vi "Minimal AR Example.vi"() -> ()   [LabVIEW 2020, in "examples.lvlib"]
doc: "Demonstrate a minimal Augmented Reality Application which Captures from a Camera, Detects AprilTags and Overlays 3D Objects on the live Camera stream."
uses:
  examples.lvlib
  ar/tvec.ctl
  ar/Roll-Pitch-Yaw.ctl
  feature_detection/Apriltag Detector/Detector Settings.ctl
  capture/Stream/Stream.lvclass/Stream.ctl
  common/Camera Parameters.ctl
  common/Camera Matrix.ctl
  common/Camera Distortion Coefficients.ctl
  feature_detection/Apriltag Detector/AprilTag Detector.lvclass/AprilTag Detector.ctl
  image/ARGB Colour.ctl
  feature_detection/Apriltag Detector/Create (Tag36h11).vi
  image/New Image (Greyscale Preallocated).vi
  image/New Image (ARGB Preallocated).vi
  capture/Stream/Next Capture (ARGB).vi
  ar/Solve PnP (IPPE Square).vi
  image/Draw Filled Poly (ARGB).vi
  image/Draw Image to Picture (ARGB).vi
  image/New Image (Greyscale Preallocated).vi/6598b9e0-8a08-46f5-91fd-ca1b87217137.vi
  image/New Image (ARGB Preallocated).vi/3321fa97-f432-4e1e-8db9-a0df79aed21b.vi
  image/ARGB Colour to U32 Pixel Value.vi
  capture/Stream/Next Capture (ARGB).vi/66171ef0-1d22-3fc5-88a4-b174a611e83f.vi
  image/ARGBExtractChannel.vi
  ar/SolvePnPCore.vi
  ar/Build Square Marker Object Points.vi
  ar/Rodrigues.vi
  ar/Rodrigues (RVec To RMat).vi
  ar/Transform Components to Transformation Matrix.vi
  image/Draw Filled Poly (ARGB).vi/e24a04ad-8575-4d64-b8af-da4c51ecb9cd.vi
  ar/Project Points.vi
  image/Draw Line (ARGB).vi
  image/Draw Image to Picture (ARGB).vi/8cd07b1b-062e-4fe4-9e87-2eb3dc89fe0e.vi
  image/Draw Line (ARGB).vi/85aa1280-0fac-47da-ba54-33850455c996.vi
  feature_detection/Apriltag Detector/CreateDetector.vi
  <vilib>/Utility/error.llb/Error Cluster From Error Code.vi
  <vilib>/Analysis/Matrix/Numeric/Conversions/Array To Matrix.vi
  <vilib>/Analysis/Matrix/Numeric/Conversions/Array To Matrix - RA2.vi
  image/image.lvlib
  capture/capture.lvlib
  capture/Stream/Stream.lvclass
  common/common.lvlib
  feature_detection/Apriltag Detector/AprilTag Detector.lvclass
  ar/ar.lvlib
panel:
  in  "Rendering":enum16{"Project Points", "3D Engine"}(ring)
  in  "Stop":bool
  out "Picture":picture
  out "Poses":T3(array[cluster]) caption="Marker Poses"
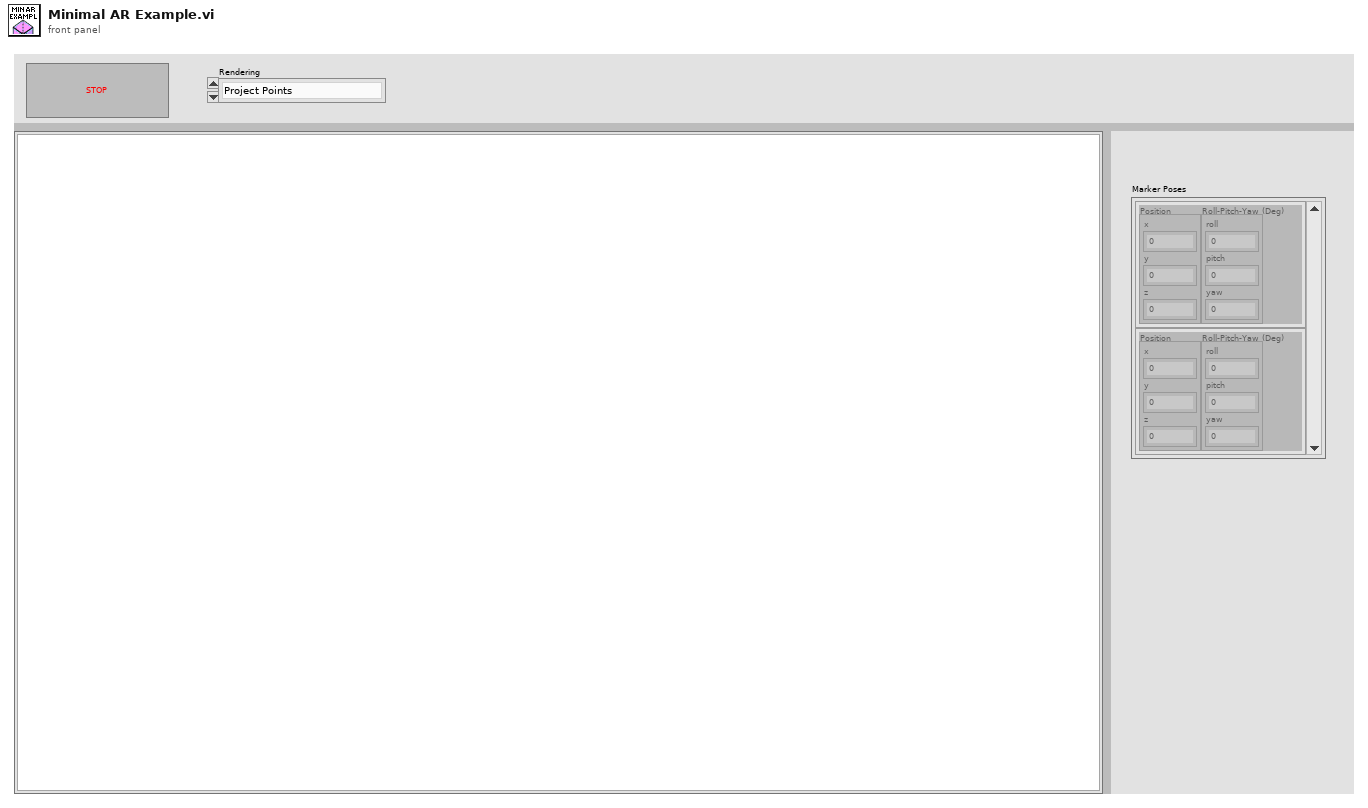
[diagram p1: front panel]
types:
  T1 = typedef "ar.lvlib/tvec.ctl" = cluster{"x":dbl, "y":dbl, "z":dbl}
  T2 = typedef "ar.lvlib/Roll-Pitch-Yaw.ctl" = cluster{"roll":dbl, "pitch":dbl, "yaw":dbl}
  T3 = cluster{"Position":T1, "Roll-Pitch-Yaw (Deg)":T2}[]
  T4 = typedef "feature_detection.lvlib/AprilTag Detector.lvclass/Detector Settings.ctl" = cluster{"Refine Edges (Default: True)":bool, "Threads (Default: 1)":u8, "Decimate (Default: 1)":sgl, "Blur (Default: 0)":sgl, "Bits (Default: 2)":u8}
  T5 = typedef "capture.lvlib/Stream.lvclass/Stream Specification.ctl" = cluster{"Size":T6, "FPS":T7}
  T6 = typedef "common.lvlib/Image Size (Integer).ctl" = cluster{"Width":u16, "Height":u16}
  T7 = typedef "capture.lvlib/Stream.lvclass/Frames per Second.ctl" = cluster{"Numerator":u32, "Denominator":u32}
  T8 = cluster{"ID":string, "Name":string, "Stream Specifications":T5[]}[]
  T9 = cluster{"ID":string, "Name":string, "Stream Specifications":T5[]}
  T10 = typedef "image.lvlib/Image Draw Offset.ctl" = cluster{"Left":i16, "Top":i16}
  T11 = typedef "common.lvlib/Camera Parameters.ctl" = cluster{"Matrix":T12, "Distortion":T13}
  T12 = typedef "common.lvlib/Camera Matrix.ctl" = cluster{"m 0,0":dbl, "m 0,1":dbl, "m 0,2":dbl, "m 1,0":dbl, "m 1,1":dbl, "m 1,2":dbl, "m 2,0":dbl, "m 2,1":dbl, "m 2,2":dbl}
  T13 = typedef "common.lvlib/Camera Distortion Coefficients.ctl" = cluster{"k1":dbl, "k2":dbl, "p1":dbl, "p2":dbl, "k3":dbl, "k4":dbl, "k5":dbl, "k6":dbl, "s1":dbl, "s2":dbl, "s3":dbl, "s4":dbl, "tau x":dbl, "tau y":dbl}
  T14 = typedef "image.lvlib/Greyscale Image.ctl" = refnum<data-value>
  T15 = typedef "image.lvlib/ARGB Image.ctl" = refnum<data-value>
  T16 = typedef "image.lvlib/ARGB Colour.ctl" = cluster{"Alpha":u8, "RGB":u32}
  T17 = typedef "feature_detection.lvlib/AprilTag Detector.lvclass/Detection.ctl" = cluster{"ID":i32, "Hamming":i32, "Decision Margin":sgl, "Centre":T18, "Corners":T19}
  T18 = typedef "common.lvlib/Image Point (Float).ctl" = cluster{"x":dbl, "y":dbl}
  T19 = typedef "common.lvlib/Quad Corners.ctl" = cluster{"Bottom Left":T18, "Bottom Right":T18, "Top Right":T18, "Top Left":T18}
  T20 = typedef "ar.lvlib/Pose.ctl" = cluster{"rvec":T21, "tvec":T1}
  T21 = typedef "ar.lvlib/rvec.ctl" = cluster{"v0":dbl, "v1":dbl, "v2":dbl}
  T22 = typedef "NI_Matrix.lvlib/RealMatrix.ctl" = dbl[][]
  T23 = typedef "ar.lvlib/Quaternion.ctl" = cluster{"w":dbl, "x":dbl, "y":dbl, "z":dbl}
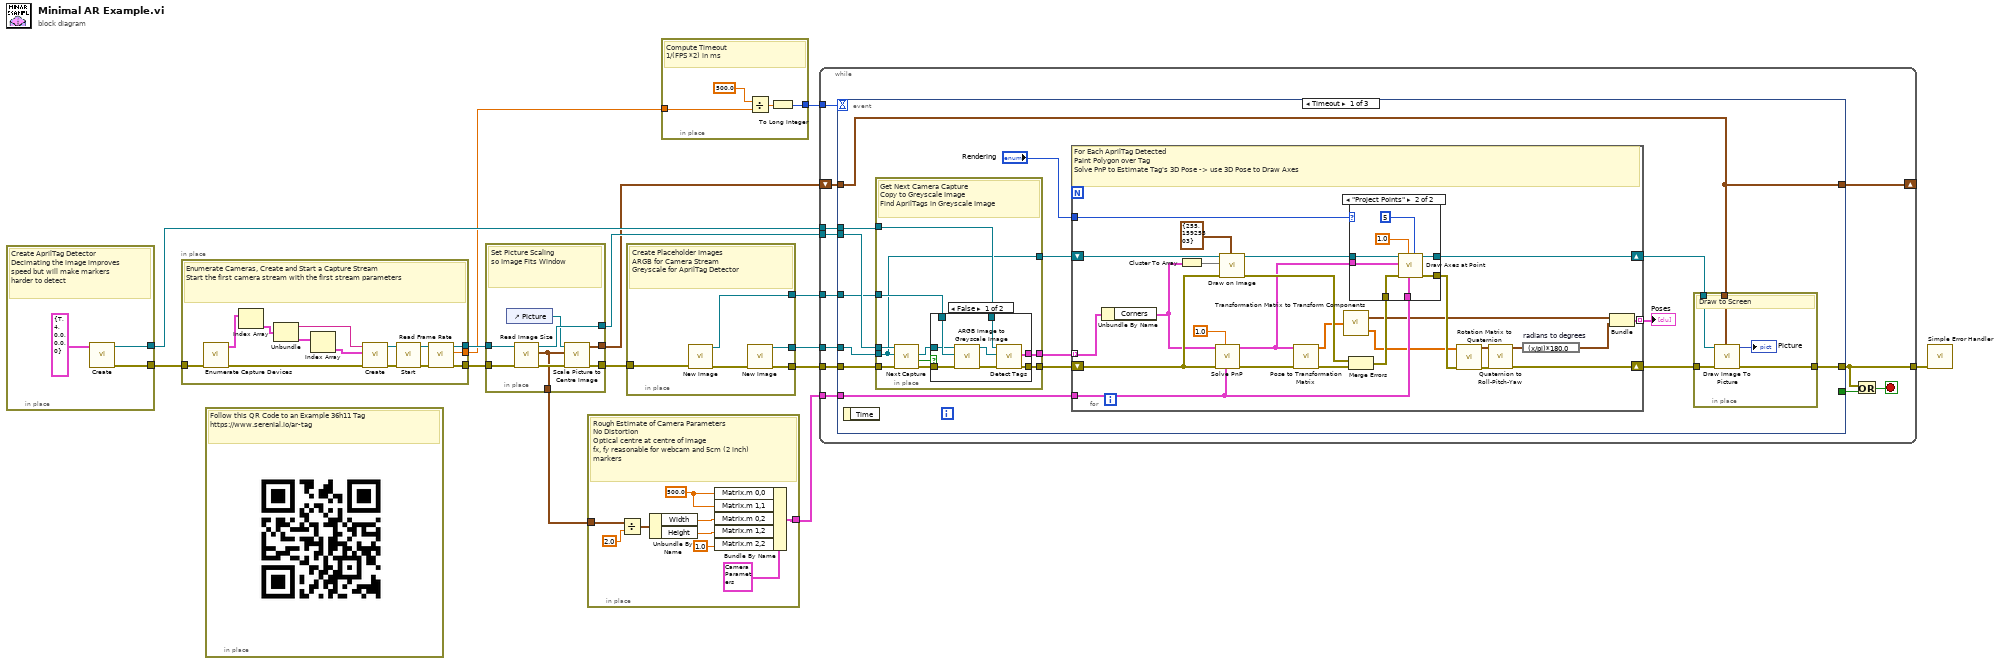
[diagram p0: block diagram]
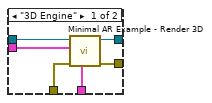
[diagram p2: hidden frame]
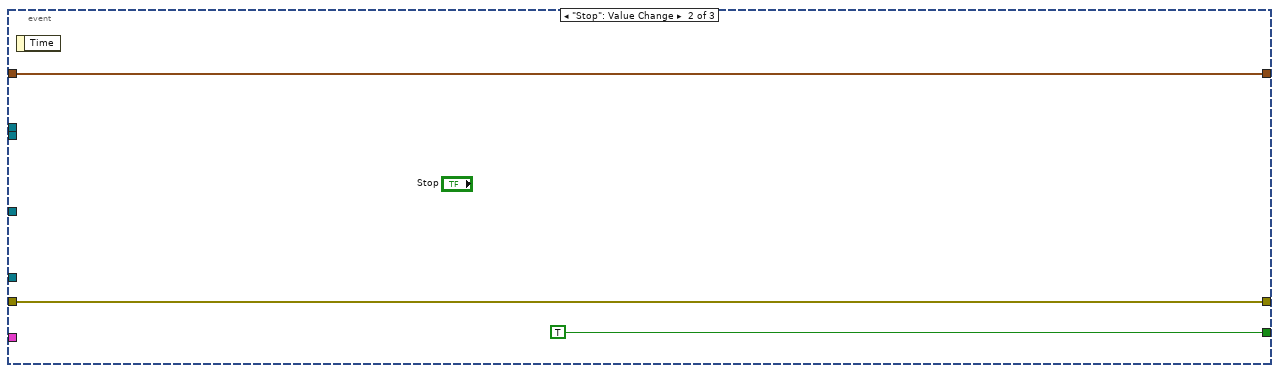
[diagram p4: hidden frame]
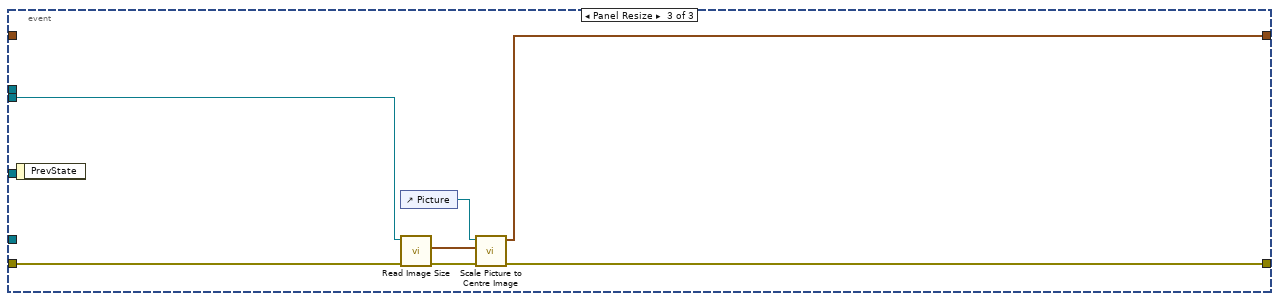
[diagram p5: hidden frame]
diagram:
  n1 = in-place {
    in-place-border: [w17] -> w9
    in-place-border: [w16] -> w7
    # "Create AprilTag Detector\nDecimating the image improves speed but will make markers\nharder to detect"
    n2 = call-poly "Create.vi"("Detector Settings"=T4 {"Refine Edges (Default: True)"=TRUE, "Threads (Default: 1)"=4, "Decimate (Default: 1)"=0.0, "Blur (Default: 0)"=0.0, "Bits (Default: 2)"=0}) -> ("error out"=w17:errorcluster, "Apriltag Detector"=w16:refnum<class "AprilTag Detector.lvclass">)  [unwired: 9 in]
  }
  n3 = in-place {
    in-place-border: [w20] -> w5
    in-place-border: [w22] -> w8
    in-place-border: w9 -> [w26]
    in-place-border: [w19] -> w2
    # "Enumerate Cameras, Create and Start a Capture Stream\nStart the first camera stream with the first stream parameters"
    n4 = call "Enumerate Capture Devices.vi"("error in (no error)"=w26) -> ("error out"=w32:errorcluster, "Devices"=w29:T8)  [unwired: 9 in]
    n5 = Index Array(array=w29) -> (element=w27:T9)  [unwired: 1 in]
    n6 = Unbundle(w27) -> ("ID"=w25:string, "Stream Specifications"=w24:T5[])  [unwired: 1 out]
    n7 = Index Array(array=w24) -> (element=w23:T5)  [unwired: 1 in]
    n8 = call "Create.vi"("error in (no error)"=w32, "Desired Stream Specification"=w23, "Device ID"=w25) -> ("error out"=w31:errorcluster, "Stream"=w30:refnum<class "Stream.lvclass">)  [unwired: 7 in]
    n9 = call "Start.vi"("error in (no error)"=w31, "Stream in"=w30) -> ("error out"=w28:errorcluster, "Stream"=w21:refnum<class "Stream.lvclass">)  [unwired: 8 in]
    n10 = call "Read Frame Rate.vi"("error in (no error)"=w28, "Stream in"=w21) -> ("error out"=w22:errorcluster, "Frame Rate (FPS)"=w19:dbl, "Stream"=w20:refnum<class "Stream.lvclass">)  [unwired: 7 in]
  }
  n11 = in-place {
    # "Follow this QR Code to an Example 36h11 Tag\nhttps://www.serenial.io/ar-tag"
  }
  n12 = in-place {
    in-place-border: w8 -> [w40]
    in-place-border: [w39] -> w6
    in-place-border: w5 -> [w37]
    in-place-border: [w36] -> w4
    in-place-border: [w35] -> w3
    in-place-border: [w33] -> w1
    # "Set Picture Scaling \nso Image Fits Window"
    n13 = control-ref of="Picture"() -> (w34:refnum<vi>)
    n14 = call "Read Image Size.vi"("error in (no error)"=w40, "Stream in"=w37) -> ("error out"=w38:errorcluster, "Image Size"=w33:T6, "Stream"=w36:refnum<class "Stream.lvclass">)  [unwired: 7 in]
    n15 = call "Scale Picture to Centre Image.vi"("error in (no error)"=w38, "Image Size"=w33, "Picture in"=w34) -> ("error out"=w39:errorcluster, "Draw Image to Picture Offset"=w35:T10)  [unwired: 6 in, 1 out]
  }
  n16 = in-place {
    in-place-border: [w42] -> w15
    in-place-border: w1 -> [w41]
    w48 = 500.0 ("Matrix.m 0,0")
    # "Rough Estimate of Camera Parameters\nNo Distortion\nOptical centre at centre of image\nfx, fy reasonable for webcam and 5cm (2 inch) markers"
    n17 = Divide(x=w41, y=2.0) -> (x/y=w46:cluster{"Width":dbl, "Height":dbl})
    n18 = Unbundle By Name(w46) -> ("Width"=w47:dbl, "Height"=w44:dbl)
    n19 = Bundle By Name(cluster=T11 {"Matrix"={"m 0,0"=0.0, "m 0,1"=0.0, "m 0,2"=0.0, "m 1,0"=0.0, "m 1,1"=0.0, "m 1,2"=0.0, "m 2,0"=0.0, "m 2,1"=0.0, "m 2,2"=0.0}, "Distortion"={"k1"=0.0, "k2"=0.0, "p1"=0.0, "p2"=0.0, "k3"=0.0, "k4"=0.0, "k5"=0.0, "k6"=0.0, "s1"=0.0, "s2"=0.0, "s3"=0.0, "s4"=0.0, "tau x"=0.0, "tau y"=0.0}} ("Camera Parameters"), "Matrix.m 0,0"=w48, "Matrix.m 1,1"=w48, "Matrix.m 0,2"=w47, "Matrix.m 1,2"=w44, "Matrix.m 2,2"=1.0) -> (w42:T11)
  }
  n20 = in-place {
    in-place-border: [w54] -> w12
    in-place-border: [w53] -> w11
    in-place-border: [w51] -> w10
    in-place-border: w6 -> [w50]
    # "Create Placeholder Images\nARGB for Camera Stream\nGreyscale for AprilTag Detector"
    n21 = call-poly "New Image.vi"("error in (no error)"=w50) -> ("error out"=w52:errorcluster, "Greyscale Image"=w53:T14)  [unwired: 9 in]
    n22 = call-poly "New Image.vi"("error in (no error)"=w52) -> ("error out"=w51:errorcluster, "ARGB Image"=w54:T15)  [unwired: 9 in]
  }
  n23 = in-place {
    in-place-border: [w56] -> w13
    in-place-border: w2 -> [w55]
    # "Compute Timeout\n1/(FPS *2) in ms"
    n24 = Divide(x=500.0 ("y"), y=w55) -> (x/y=w57:dbl)
    n25 = To Long Integer(number=w57) -> (32bit integer=w56:i32)
  }
  n26 = while {
    tunnel: w10 -> [w70]
    tunnel: [w67] -> w14
    tunnel: w12 -> [w66]
    tunnel: w11 -> [w65]
    tunnel: w7 -> [w64]
    tunnel: w15 -> [w63]
    tunnel: w4 -> [w69]
    tunnel: w13 -> [w61]
    shift-right: [w59] -> _
    shift-left: w3 -> [w60]
    stop <- w68 stop-if-true
    n27 = event shown="[0] Timeout" {
      selector: _ -> [_ _ _]
      dyn-events: _ -> [_ _ _]
      timeout: w61 -> [_ _ _]
      tunnel: w70 -> [w85 w151 w159]
      tunnel: w69 -> [w84 _ w158]
      tunnel: [w83 w151 w153] -> w67
      tunnel: w66 -> [w82 _ _]
      tunnel: w65 -> [w81 _ _]
      tunnel: w64 -> [w80 _ _]
      tunnel: w63 -> [w74 _ _]
      tunnel: [_ TRUE _] -> w62
      tunnel: w60 -> [w73 w150 _]
      tunnel: [w73 w150 w154] -> w59
      event Timeout {
        n28 = event-data() -> ()  [unwired: 1 in, 1 out]
        n29 = in-place {
          in-place-border: w85 -> [w135]
          in-place-border: w84 -> [w134]
          in-place-border: w82 -> [w128]
          in-place-border: w81 -> [w133]
          in-place-border: w80 -> [w131]
          in-place-border: [w130] -> w79
          in-place-border: [w129] -> w77
          in-place-border: [w128] -> w76
          # "Get Next Camera Capture\nCopy to Greyscale Image\nFind AprilTags in Greyscale Image"
          n30 = call-poly "Next Capture.vi"("error in (no error)"=w135, "ARGB Destination Image in"=w128, "Stream in"=w134) -> ("error out"=w132:errorcluster, "Timed Out?"=w127:bool, "ARGB Destination Image"=w126:T15)  [unwired: 5 in, 1 out]
          n31 = case shown="False" w127 {
            tunnel: w133 -> [w143 _]
            tunnel: w132 -> [w142 w144]
            tunnel: w131 -> [w141 _]
            tunnel: [w140 w144] -> w130
            tunnel: [w139 _] -> w129
            tunnel: w126 -> [w138 _]
            frame False {
              n32 = call "ARGB Image to Greyscale Image.vi"("error in (no error)"=w142, "Greyscale Image Destination in"=w143, "ARGB Image Source in"=w138) -> ("error out"=w137:errorcluster, "Greyscale Image Destination"=w136:T14)  [unwired: 7 in]
              n33 = call "Detect Tags.vi"("error in (no error)"=w137, "Greyscale Image in"=w136, "Apriltag Detector in"=w141) -> ("error out"=w140:errorcluster, "Detections"=w139:T17[])  [unwired: 5 in, 2 out]
            }
            frame True {
            }
          }
        }
        n34 = for {
          tunnel: w77 -> [w104] mode=indexing
          tunnel: w74 -> [w100]
          shift-right: [w96] -> w78
          shift-left: w79 -> [w109]
          shift-right: [w101] -> w75
          shift-left: w76 -> [w108]
          tunnel: "Rendering" -> [w99]
          tunnel: [w93] -> w71 mode=indexing
          # "For Each AprilTag Detected\nPaint Polygon over Tag\nSolve PnP to Estimate Tag's 3D Pose -> use 3D Pose to Draw Axes"
          n35 = Unbundle By Name(w104) -> ("Corners"=w90:T19)
          n36 = Cluster To Array(cluster=w90) -> (array=w107:T18[])
          n37 = call-poly "Solve PnP.vi"("Camera Parameters"=w100, "Square Length"=1.0, "error in (no error)"=w109, "Square Corners"=w90) -> ("error out"=w88:errorcluster, "Pose"=w87:T20)  [unwired: 6 in]
          n38 = call-poly "Draw on Image.vi"("ARGB Colour"=T16 {"Alpha"=255, "RGB"=15925503}, "error in (no error)"=w109, "Points"=w107, "ARGB Image in"=w108) -> ("error out"=w110:errorcluster, "ARGB Image"=w103:T15)  [unwired: 6 in]
          n39 = call "Pose to Transformation Matrix.vi"("error in (no error)"=w88, "Pose"=w87) -> ("error out"=w86:errorcluster, "4x4 Transformation Matrix"=w89:T22)  [unwired: 8 in]
          n40 = call "Transformation Matrix to Transform Components.vi"("4x4 Transformation Matrix"=w89) -> ("tvec"=w91:T1, "Rotation Matrix"=w92:T22)
          n41 = Merge Errors(w110, w86) -> (w102:errorcluster)
          n42 = case shown="\"Project Points\"" w99 {
            tunnel: w103 -> [w116 w125]
            tunnel: w102 -> [w117 w124]
            tunnel: [w115 w123] -> w101
            tunnel: [w114 w122] -> w111
            tunnel: w100 -> [w113 w119]
            tunnel: w87 -> [w112 w118]
            frame "3D Engine" {
              n43 = call "Minimal AR Example - Render 3D.vi"("Camera Parameters"=w113, "error in (no error)"=w117, "Pose"=w112, "ARGB Image In"=w116) -> ("error out"=w114:errorcluster, "ARGB Image Out"=w115:T15)  [unwired: 6 in]
            }
            frame "Project Points" {
              n44 = call "Draw Axes at Point.vi"("Thickness (Default: 1)"=5, "Camera Parameters"=w119, "Length"=1.0, "error in (no error)"=w124, "Pose"=w118, "ARGB Image in"=w125) -> ("error out"=w122:errorcluster, "ARGB Image"=w123:T15)  [unwired: 4 in]
            }
          }
          n45 = call "Rotation Matrix to Quaternion.vi"("error in (no error)"=w111, "Rotation Matrix"=w92) -> ("error out"=w98:errorcluster, "Quaternion"=w97:T23)  [unwired: 8 in]
          n46 = call "Quaternion to Roll-Pitch-Yaw.vi"("error in (no error)"=w98, "Quaternion"=w97) -> ("error out"=w96:errorcluster, "Roll-Pitch-Yaw (rad)"=w95:T2)  [unwired: 8 in]
          n47 = expression code="(x/pi)*180.0" "radians to degrees"(w95) -> (w94:T2)
          n48 = Bundle("tvec"=w91, "Roll-Pitch-Yaw (rad)"=w94) -> (w93:cluster{"tvec":T1, "Roll-Pitch-Yaw (rad)":T2})  [unwired: 1 in]
        }
        "Poses" <- w71
        n49 = in-place {
          in-place-border: [w148] -> w83
          in-place-border: w78 -> [w147]
          in-place-border: w75 -> [w146]
          in-place-border: w73 -> [w145]
          # "Draw to Screen"
          n50 = call-poly "Draw Image To Picture.vi"("Image Draw Offset (Default 0,0)"=w145, "error in (no error)"=w147, "ARGB Image Source in"=w146) -> ("error out"=w148:errorcluster, "Picture"=→"Picture":picture)  [unwired: 7 in]
        }
      }
      event "Stop": Value Change {
        n51 = event-data() -> ()  [unwired: 1 in, 1 out]
      }
      event Panel Resize {
        n52 = event-data() -> ()  [unwired: 1 in, 1 out]
        n53 = control-ref of="Picture"() -> (w156:refnum<vi>)
        n54 = call "Read Image Size.vi"("error in (no error)"=w159, "Stream in"=w158) -> ("error out"=w157:errorcluster, "Image Size"=w155:T6)  [unwired: 7 in, 1 out]
        n55 = call "Scale Picture to Centre Image.vi"("error in (no error)"=w157, "Image Size"=w155, "Picture in"=w156) -> ("error out"=w153:errorcluster, "Draw Image to Picture Offset"=w154:T10)  [unwired: 6 in, 1 out]
      }
    }
    n56 = Or(x=w67, y=w62) -> (x .or. y?=w68:bool)
  }
  n57 = call <vilib>:"Simple Error Handler.vi"("error in (no error)"=w14) -> ()  [unwired: 4 in, 5 out]
